vi "Controller Algorithm.vi"(8 "Heater Output":refnum<class "Abs_Boolean.lvclass">, 9 "Lower Limit":refnum<class "Abs_Double Float.lvclass">, 10 "Upper Limit":refnum<class "Abs_Double Float.lvclass">, 11 "Reading":refnum<class "Abs_Double Float.lvclass">) -> (3 "Node Out":refnum<class "bt_Node.lvclass">)   [LabVIEW 2021]
uses:
  Support/Nodes/abs_Node/bt_Node.lvclass
  <vilib>/TSA/Abstract Data Classes/Abs_Types/Double Float/Abs_Double Float.lvclass
  C:/Program Files (x86)/National Instruments/LabVIEW 2021/vi.lib/TSA/Abstract Data Classes/Abs_Types/Numeric/Abs_Numeric.lvclass
  <vilib>/TSA/Abstract Data Classes/Abs_Types/Boolean/Abs_Boolean.lvclass
  C:/Program Files (x86)/National Instruments/LabVIEW 2021/vi.lib/TSA/Abstract Data Classes/Abs_Types/Value/Abs_Value.lvclass
  C:/Program Files (x86)/National Instruments/LabVIEW 2021/vi.lib/TSA/Abstract Data Classes/Abs_Types/Type/Abs_Type.lvclass
  Support/Nodes/Leaves/abs_Type Leaf/abs_Type Leaf.lvclass/abs_Type Leaf.ctl
  Support/Nodes/Leaves/abs_Type Leaf/Properties/Write Value Class.vi
  Support/Nodes/Leaves/Test Boolean/Test Abs_Boolean.lvclass
  C:/Users/Tim/Documents/GitHub/LV_Behaviour_Tree/Source/Support/Nodes/abs_Node/bt_Node.lvclass
  C:/Users/Tim/Documents/GitHub/LV_Behaviour_Tree/Source/Support/Nodes/Leaves/abs_Type Leaf/abs_Type Leaf.lvclass
  <vilib>/TSA/Abstract Data Classes/Functions/Compare/Support/Greater/DBL/Method.vi
  <vilib>/TSA/Abstract Data Classes/Functions/Compare/Support/Less/DBL/Method.vi
  <vilib>/TSA/Abstract Data Classes/Constants/Support/Bool/Bool.vi
  BT.lvlib
  <vilib>/TSA/Abstract Data Classes/Functions/Compare/Support/Less/DBL/Less_DBL.lvclass
  C:/Program Files (x86)/National Instruments/LabVIEW 2021/vi.lib/TSA/Abstract Data Classes/Abs_Types/Floating Point/Abs_Floating Point.lvclass
  C:/Program Files (x86)/National Instruments/LabVIEW 2021/vi.lib/TSA/Abstract Data Classes/Abs_Types/Double Float/Abs_Double Float.lvclass
  <vilib>/TSA/Abstract Data Classes/Functions/Compare/Support/Greater/DBL/Greater_DBL.lvclass
  <vilib>/TSA/Abstract Data Classes/Constants/Support/Bool/Const_Bool.lvclass
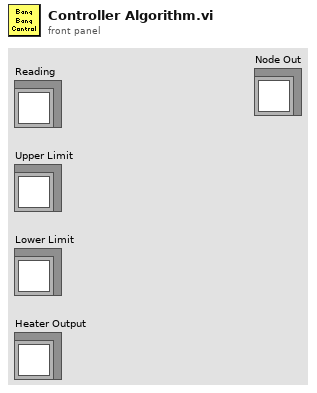
[diagram p1: front panel]
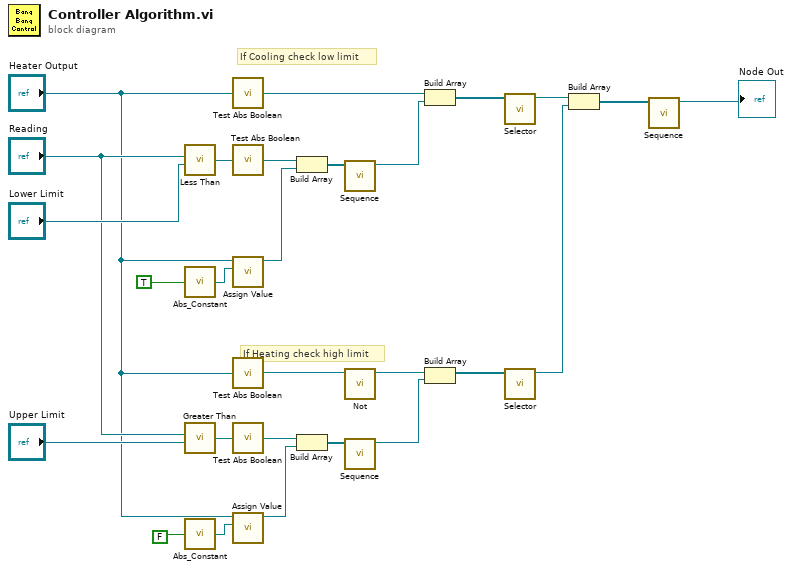
[diagram p0: block diagram]
diagram:
  # "If Heating check high limit"
  # "If Cooling check low limit"
  n1 = call-poly <vilib>:"Less Than.vi"("Value B"="Lower Limit", "Value A"="Reading") -> ("Result"=w13:refnum<class "Abs_Boolean.lvclass">)  [unwired: 4 in]
  n2 = call-poly <vilib>:"Abs_Constant.vi"("Boolean"=TRUE ("Boolean Value")) -> ("Abs_Boolean.lvclass"=w5:refnum<class "Abs_Boolean.lvclass">)  [unwired: 4 in]
  n3 = call-poly <vilib>:"Greater Than.vi"("Value B"="Upper Limit", "Value A"="Reading") -> ("Result"=w9:refnum<class "Abs_Boolean.lvclass">)  [unwired: 4 in]
  n4 = call-poly <vilib>:"Abs_Constant.vi"("Boolean"=FALSE ("Boolean Value")) -> ("Abs_Boolean.lvclass"=w2:refnum<class "Abs_Boolean.lvclass">)  [unwired: 4 in]
  n5 = call "Test Abs Boolean.vi"("Abs_Boolean.lvclass"="Heater Output") -> ("abs_Node"=w17:refnum<class "bt_Node.lvclass">)  [unwired: 4 in]
  n6 = call "Test Abs Boolean.vi"("Abs_Boolean.lvclass"=w13) -> ("abs_Node"=w14:refnum<class "bt_Node.lvclass">)  [unwired: 4 in]
  n7 = call "Assign Value.vi"("Assigned Value"=w5, "Value"="Heater Output") -> ("Node Out"=w4:refnum<class "bt_Node.lvclass">)  [unwired: 9 in]
  n8 = call "Test Abs Boolean.vi"("Abs_Boolean.lvclass"="Heater Output") -> ("abs_Node"=w16:refnum<class "bt_Node.lvclass">)  [unwired: 4 in]
  n9 = call "Test Abs Boolean.vi"("Abs_Boolean.lvclass"=w9) -> ("abs_Node"=w8:refnum<class "bt_Node.lvclass">)  [unwired: 4 in]
  n10 = call "Assign Value.vi"("Assigned Value"=w2, "Value"="Heater Output") -> ("Node Out"=w6:refnum<class "bt_Node.lvclass">)  [unwired: 9 in]
  n11 = Build Array(w14, w4) -> (w26:refnum<class "bt_Node.lvclass">[])
  n12 = Build Array(w8, w6) -> (w21:refnum<class "bt_Node.lvclass">[])
  n13 = call "Sequence.vi"("Nodes"=w26) -> ("Node"=w25:refnum<class "bt_Node.lvclass">)  [unwired: 10 in]
  n14 = call "Not.vi"("Node In"=w16) -> ("Node"=w15:refnum<class "bt_Node.lvclass">)  [unwired: 10 in]
  n15 = call "Sequence.vi"("Nodes"=w21) -> ("Node"=w22:refnum<class "bt_Node.lvclass">)  [unwired: 10 in]
  n16 = Build Array(w17, w25) -> (w27:refnum<class "bt_Node.lvclass">[])
  n17 = Build Array(w15, w22) -> (w19:refnum<class "bt_Node.lvclass">[])
  n18 = call "Selector.vi"("Nodes"=w27) -> ("Node"=w24:refnum<class "bt_Node.lvclass">)  [unwired: 10 in]
  n19 = call "Selector.vi"("Nodes"=w19) -> ("Node"=w18:refnum<class "bt_Node.lvclass">)  [unwired: 10 in]
  n20 = Build Array(w24, w18) -> (w23:refnum<class "bt_Node.lvclass">[])
  n21 = call "Sequence.vi"("Nodes"=w23) -> ("Node"=→"Node Out":refnum<class "bt_Node.lvclass">)  [unwired: 10 in]
